vi "Set Message Transport AF Enqueuer.vi"(8 "error in (no error)":errorcluster, 10 "Message AF Mediator":refnum<class "Message AF Mediator.lvclass">, 11 "Actor's Enqueuer":refnum<class "Message Enqueuer.lvclass">) -> (0 "error out":errorcluster, 3 "Message Transport Actor Framework out":refnum<class "Message Transport Actor Framework.lvclass">)   [LabVIEW 2016, in "Stream Mediator.lvlib" / "Message Transport Actor Framework.lvclass"]
doc: "--\nCopyright © 2017 Composed SystemsI All rights reserved.\n\nAuthor: Jon McBee <jon.mcbee@composed.io>\n\nThis library is provided \"AS IS\" ,WITHOUT WARRANTIES OR\nCONDITIONS OF ANY KIND, either express or implied.\n\nComposed Systems -- composed.io\n\nStream 0.0.1.1\nJon McBee - Composed Systems\nCopyright (c) 2017, Composed Systems"
uses:
  <userlib>/Composed Systems/Stream/Mediator/Classes/Message Transport Actor Framework/Message Transport Actor Framework.lvclass
  <vilib>/ActorFramework/Message Enqueuer/Message Enqueuer.lvclass
  <userlib>/Composed Systems/Stream/Mediator/Classes/Message AF Mediator/Message AF Mediator.lvclass
  <userlib>/Composed Systems/Stream/Mediator/Classes/Message Transport Actor Framework/Message Transport Actor Framework.lvclass/Message Transport Actor Framework.ctl
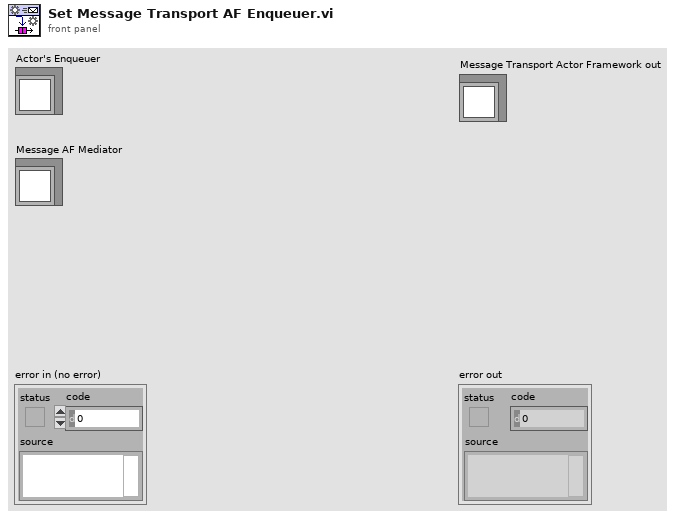
[diagram p1: front panel]
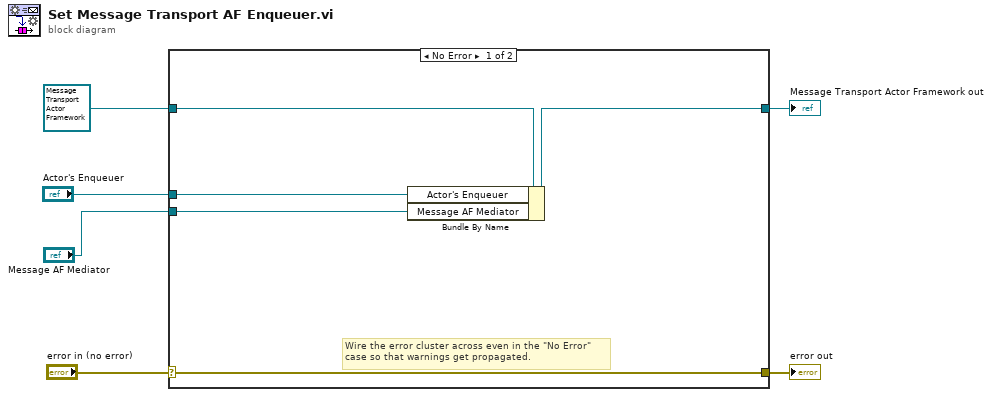
[diagram p0: block diagram]
diagram:
  n1 = case shown="No Error" "error in (no error)" {
    selector: "error in (no error)" -> [w11 w13]
    tunnel: [w11 w13] -> w5
    tunnel: [w9 w12] -> w3
    tunnel: refnum<class "Message Transport Actor Framework.lvclass"> refnum ("Message Transport Actor Framework in") -> [w10 w12]
    tunnel: "Actor's Enqueuer" -> [w8 _]
    tunnel: "Message AF Mediator" -> [w7 _]
    frame No Error {
      # "Wire the error cluster across even in the \"No Error\"\ncase so that warnings get propagated."
      n2 = Bundle By Name(cluster=w10, "Actor's Enqueuer"=w8, "Message AF Mediator"=w7) -> (w9:refnum<class "Message Transport Actor Framework.lvclass">)
    }
    frame Error {
    }
  }
  "error out" <- w5
  "Message Transport Actor Framework out" <- w3
